vi "initialize.vi"(7 "action name":string, 8 "error in":errorcluster, 10 "parameters":variant, 11 "action in":refnum<class "action.lvclass">) -> (0 "error out":errorcluster, 3 "action out":refnum<class "action.lvclass">)   [LabVIEW 2013, in "action.lvclass"]
uses:
  action.lvclass
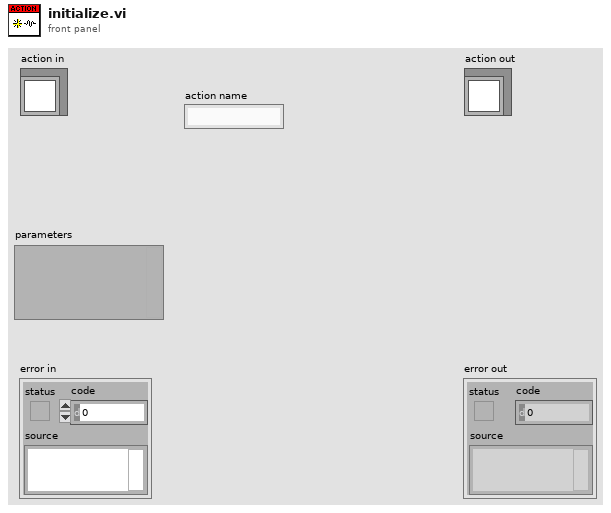
[diagram p1: front panel]
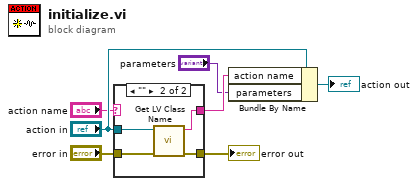
[diagram p0: block diagram]
diagram:
  n1 = case shown="\"\"" "action name" {
    selector: "action name" -> [w9 _]
    tunnel: "error in" -> [w8 w13]
    tunnel: [w8 w12] -> w5
    tunnel: "action in" -> [_ w11]
    tunnel: [w9 w10] -> w2
    frame Default {
    }
    frame "" {
      n2 = call <vilib>:"Get LV Class Name.vi"("error in (no error)"=w13, "object"=w11) -> ("error out"=w12:errorcluster, "class name"=w10:string)  [unwired: 8 in]
    }
  }
  "error out" <- w5
  n3 = Bundle By Name(cluster="action in", "action name"=w2, "parameters"="parameters") -> (→"action out":refnum<class "action.lvclass">)
